vi "Teleop.vi"(10 "Match Info":T1={"Autonomous Elapsed Seconds"=0.0, "TeleOp Elapsed Seconds"=0.0, "Disabled Elapsed Seconds"=0.0, "Visited Autonomous"=FALSE, "Visited TeleOp"=FALSE, "Visited Disabled"=FALSE, "Autonomous Settings"={"Autonomous Style"=enum."Independent", "VI Refnum"=refnum}}, 11 "Call Context":T2=enum."Stop") -> ()   [LabVIEW 2018]
doc: "This VI is called for each enabled TeleOp packet received from the DS. It is typically used to read from joysticks and other inputs and update I/O or setpoints for timed control loops. It should complete and return within 20 milliseconds or risk missing DS packets."
uses:
  <vilib>/Rock Robotics/WPI/DriverStation/WPI_DriverStationDerivedRobotMode.ctl
  <vilib>/Rock Robotics/WPI/DriverStation/WPI_DriverStationMatch Info.ctl
  Typedef/XBox Axis.ctl
  Typedef/XBox Buttons.ctl
  <vilib>/Rock Robotics/WPI/Utilities/WPI_GetSetVariantRefNum.vi
  <vilib>/Rock Robotics/Network Tables/NT Write Boolean Array.vi
  <vilib>/Rock Robotics/Network Tables/NT Write Numeric Array.vi
  <vilib>/Rock Robotics/Network Tables/NT Write Number.vi
  <vilib>/Rock Robotics/Network Tables/NT Read Number.vi
  Subsystem Sequencer/Commands/Elevator to Position.vi
  <vilib>/Rock Robotics/WPI/MotorControl/WPI_MotorControlRefNum Registry Get.vi
  <vilib>/Rock Robotics/WPI/ThirdParty/REV Robotics/SPARK MAX/SubVI/Public/Spark MAX Set Smart Motion Constraints.vi
  <vilib>/Rock Robotics/WPI/Solenoid/WPI_SolenoidRefNum Registry Get.vi
  <vilib>/Rock Robotics/WPI/Solenoid/WPI_SolenoidSet.vi
  <vilib>/Rock Robotics/WPI/Solenoid/WPI_SolenoidSetEnum.vi
  Drive/CAN Functions/CAN 6 SPARK MAX Motor Ref Get.vi
  Drive/CAN Functions/CAN 6 SPARK MAX Motor Set Idle Modes.vi
  Subsystem Sequencer/Commands/Climb Sequence Three.vi
  Subsystem Sequencer/Commands/Climb Sequence Two.vi
  Subsystem Sequencer/Commands/Climb Sequence One.vi
panel:
  in  "max queso power (1)":dbl=0.6
  in  "Limelight Speed Limit":dbl=0.5
  in  "Elevator Slow Acceleration":dbl=800.0
  in  "Elevator Slow Velocity":dbl=400.0
  in  "Arm angle from 'Y'":dbl=86.0 format="%#_13g"
  in  "Joystick Deadband":dbl=0.06 format="%#_13g"
  in  "Throttle Sensitivity":dbl(slide)=0.7142857142857142 scale=0.0..1.0
  in  "Elevator Speed":dbl=1.5 format="%#_13g"
  in  "QuesoTurn Sensitivty":dbl=0.7
  in  "Cheesy Sensitivity":dbl(slide)=0.5864661654135338 scale=0.0..1.0
  in  "Arcade to Queso":bool=TRUE
  # "<-- This is not motor speed!"
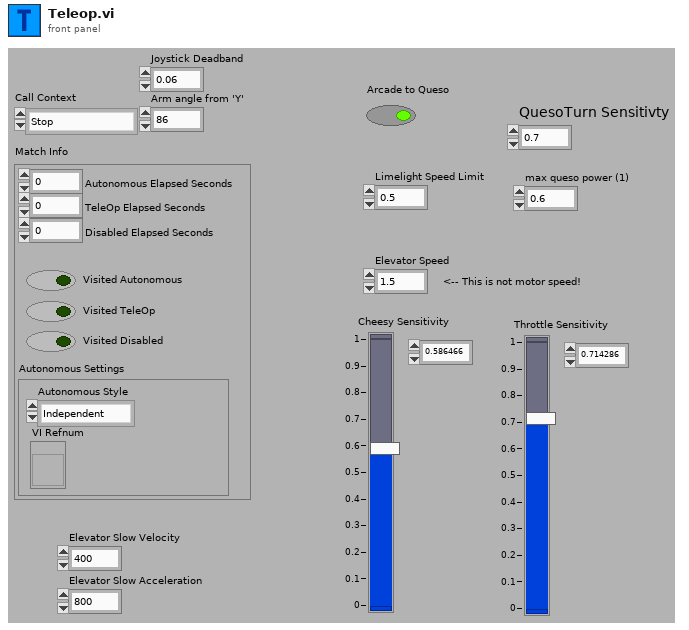
[diagram p1: front panel]
types:
  T1 = typedef "WPI_DriverStationMatch Info.ctl" = cluster{"Autonomous Elapsed Seconds":dbl, "TeleOp Elapsed Seconds":dbl, "Disabled Elapsed Seconds":dbl, "Visited Autonomous":bool, "Visited TeleOp":bool, "Visited Disabled":bool, "Autonomous Settings":cluster{"Autonomous Style":enum16{"Iterative", "Independent"}, "VI Refnum":refnum<vi>}}
  T2 = typedef "WPI_DriverStationDerivedRobotMode.ctl" = enum16{"Init", "Execute", "Stop"}
  T3 = typedef "XBox Buttons.ctl" = enum16{"A", "B", "X", "Y", "Left Bumper", "Right Bumper", "Back", "Start", "Left Joystick", "Right Joystick"}
  T4 = typedef "XBox Axis.ctl" = enum16{"Left X", "Left Y", "Left Trigger", "Right Trigger", "Right X", "Right Y"}
  T5 = typedef "WPI_JoystickDevRef.ctl" = cluster{"Device":T6}
  T6 = typedef "WPI_JoystickDeviceEnum.ctl" = enum16{"USB 0", "USB 1", "USB 2", "USB 3", "USB 4", "USB 5"}
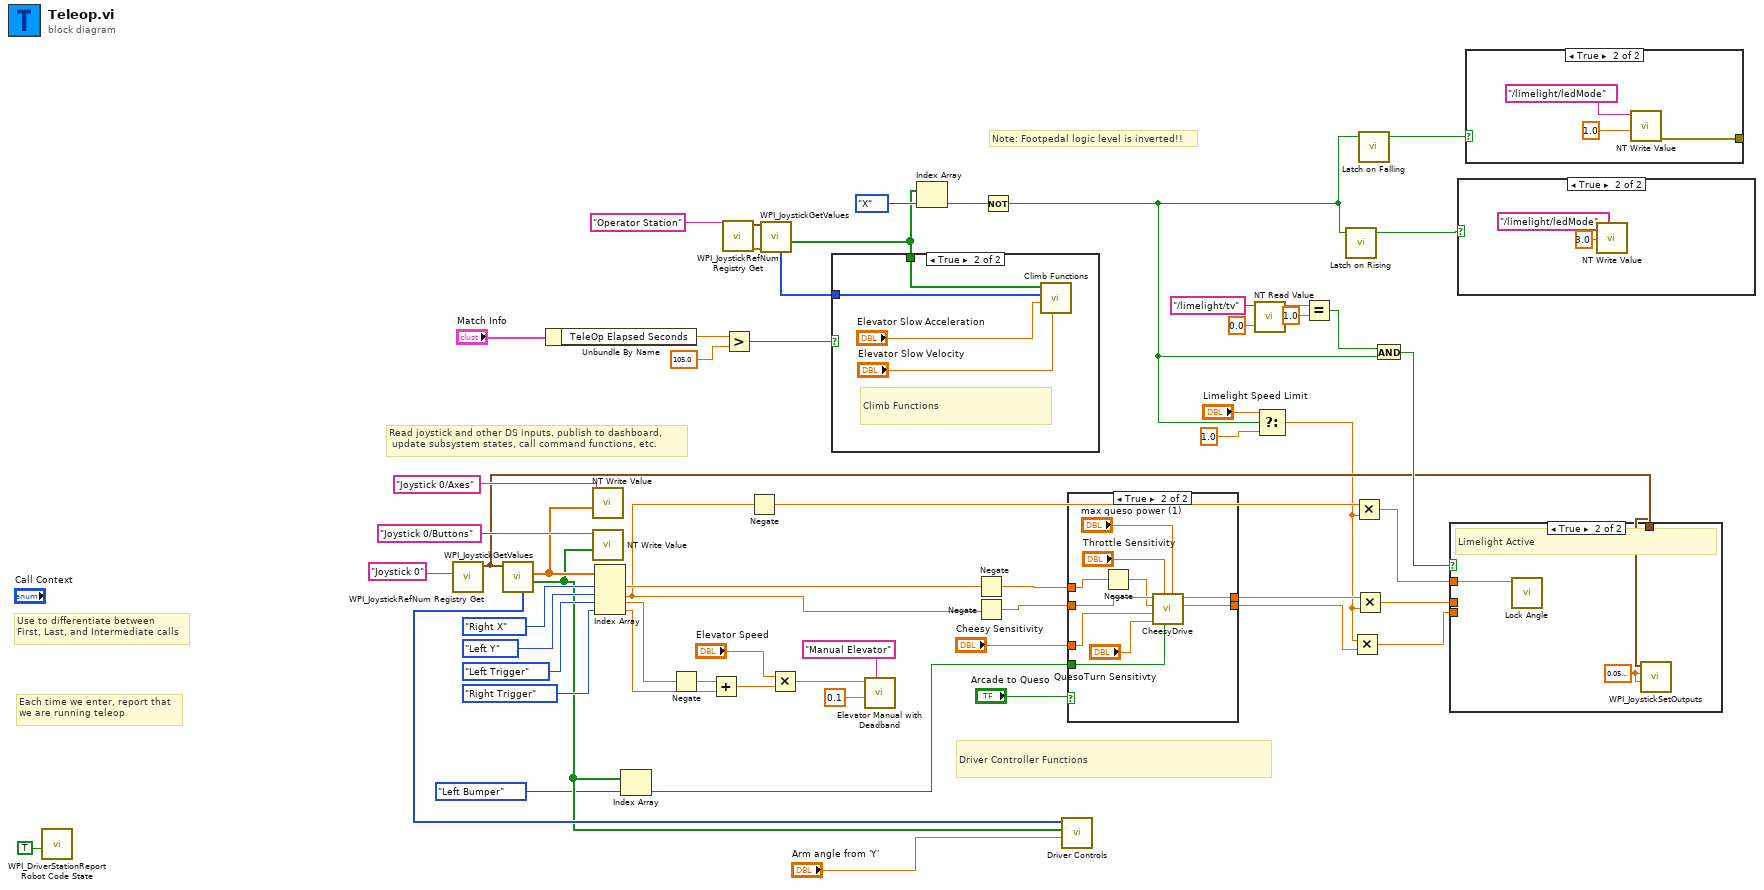
[diagram p0: block diagram]
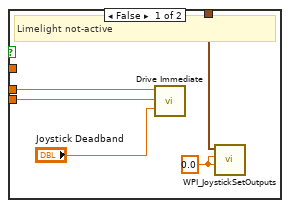
[diagram p5: hidden frame]
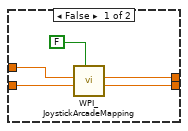
[diagram p6: hidden frame]
diagram:
  # "Driver Controller Functions"
  # "Note: Footpedal logic level is inverted!!"
  # "Read joystick and other DS inputs, publish to dashboard,\n update subsystem states, call command functions, etc."
  # "Each time we enter, report that\nwe are running teleop"
  # "Use to differentiate between\nFirst, Last, and Intermediate calls"
  n1 = call <vilib>:"WPI_DriverStationReport Robot Code State.vi"("TeleOp"=TRUE ("Autonomous")) -> ()  [unwired: 10 in, 1 out]
  n2 = call <vilib>:"WPI_JoystickRefNum Registry Get.vi"("refnum name"="Joystick 0") -> ("JoystickDevRef"=w24:T5)  [unwired: 1 in, 9 out]
  n3 = call <vilib>:"WPI_JoystickGetValues.vi"("JoystickDevRef"=w24) -> ("Buttons"=w17:bool[], "Axes"=w54:dbl[], "POVs"=w19:i16[])  [unwired: 6 in, 2 out]
  n4 = Unbundle By Name("Match Info") -> ("TeleOp Elapsed Seconds"=w3:dbl)
  n5 = call-poly <vilib>:"NT Write Value.vi"("Numeric Array"=w54, "Name"="Joystick 0/Axes") -> ()  [unwired: 9 in, 1 out]
  n6 = call-poly <vilib>:"NT Write Value.vi"("Boolean Array"=w17, "Name"="Joystick 0/Buttons") -> ()  [unwired: 9 in, 1 out]
  n7 = Index Array(array=w54, index #1=XBox_Axis."Right X" ("Enum"), index #2=XBox_Axis."Left Y" ("Enum"), index #3=XBox_Axis."Left Trigger" ("Enum"), index #4=XBox_Axis."Right Trigger" ("Enum")) -> (element #1=w50:dbl, element #2=w23:dbl, element #3=w43:dbl, element #4=w42:dbl)
  n8 = Index Array(array=w17, index=XBox_Buttons."Left Bumper" ("Enum")) -> (element=w15:bool)
  n9 = Negate(x=w43) -> (-x=w40:dbl)
  n10 = Add(x=w40, y=w42) -> (x+y=w41:dbl)
  n11 = call <vilib>:"WPI_JoystickRefNum Registry Get.vi"("refnum name"="Operator Station") -> ("error out"=w35:errorcluster, "JoystickDevRef"=w34:T5)  [unwired: 9 in]
  n12 = Greater?(x=w3, y=105.0) -> (0:w2:bool)
  n13 = Negate(x=w23) -> (-x=w8:dbl)
  n14 = call <vilib>:"WPI_JoystickGetValues.vi"("error in (no error)"=w35, "JoystickDevRef"=w34) -> ("Buttons"=w18:bool[], "POVs"=w20:i16[])  [unwired: 5 in, 3 out]
  n15 = Multiply(x="Elevator Speed", y=w41) -> (x*y=w38:dbl)
  n16 = case shown="True" w2 {
    tunnel: w20 -> [_ w62]
    tunnel: w18 -> [_ w61]
    frame False {
    }
    frame True {
      # "Climb Functions"
      n17 = call "Climb Functions.vi"("Elevator Slow Velocity"="Elevator Slow Velocity", "Elevator Slow Acceleration"="Elevator Slow Acceleration", "POVs"=w62, "Buttons"=w61) -> ()  [unwired: 8 in]
    }
  }
  n18 = call "Elevator Manual with Deadband.vi"("Description"="Manual Elevator", "Deadband Value"=0.1, "Setpoint"=w38) -> ()  [unwired: 8 in, 1 out]
  n19 = Index Array(array=w18, index=XBox_Buttons."X" ("Enum")) -> (element=w31:bool)
  n20 = Negate(x=w50) -> (-x=w48:dbl)
  n21 = Negate(x=w23) -> (-x=w49:dbl)
  n22 = Not(x=w31) -> (.not. x?=w7:bool)
  n23 = call "Driver Controls.vi"("Arm angle from 'Y'"="Arm angle from 'Y'", "Buttons"=w17, "POVs"=w19) -> ()  [unwired: 9 in]
  n24 = case shown="True" "Arcade to Queso" {
    tunnel: w49 -> [w66 w74]
    tunnel: w48 -> [w67 w73]
    tunnel: [w65 w77] -> w12
    tunnel: [w64 w76] -> w10
    tunnel: w15 -> [_ w75]
    tunnel: "Cheesy Sensitivity" -> [_ w71]
    frame False {
      n25 = call <vilib>:"WPI_JoystickArcadeMapping.vi"("Square Inputs"=FALSE, "Y axis value"=w66, "X axis value"=w67) -> ("Right Motor Value"=w65:dbl, "Left Motor Value"=w64:dbl)  [unwired: 7 in]
    }
    frame True {
      n26 = Negate(x=w73) -> (-x=w72:dbl)
      n27 = call "CheesyDrive.vi"("max queso power (1)"="max queso power (1)", "Quickturn"=w75, "Throttle Sensitivity"="Throttle Sensitivity", "QuickTurn Sensitivty"="QuesoTurn Sensitivty", "Queso Arc Sensitivty"=w71, "Wheel"=w72, "Throttle"=w74) -> ("Right PWM"=w77:dbl, "Left PWM"=w76:dbl)  [unwired: 3 in]
    }
  }
  n28 = call-poly <vilib>:"NT Read Value.vi"("Default Value"=0.0, "Name"="/limelight/tv") -> ("Numeric"=w28:dbl)  [unwired: 8 in, 1 out]
  n29 = Select(t="Limelight Speed Limit", s=w7, f=1.0) -> (s? t:f=w5:dbl)
  n30 = Equal?(x=w28, y=1.0) -> (x = y?=w26:bool)
  n31 = call "Latch on Rising.vi"("Boolean in"=w7) -> ("Boolean out"=w22:bool)  [unwired: 4 in]
  n32 = Multiply(x=w5, y=w12) -> (x*y=w13:dbl)
  n33 = Multiply(x=w8, y=w5) -> (x*y=w9:dbl)
  n34 = Multiply(x=w10, y=w5) -> (x*y=w11:dbl)
  n35 = call "Latch on Falling.vi"("Boolean in"=w7) -> ("Boolean out"=w21:bool)  [unwired: 4 in]
  n36 = And(x=w26, y=w7) -> (x .and. y?=w25:bool)
  n37 = case shown="True" w25 {
    tunnel: w13 -> [w81 _]
    tunnel: w11 -> [w80 _]
    tunnel: w9 -> [_ w85]
    tunnel: w24 -> [w79 w84]
    frame False {
      w78 = sgl 0.0 ("Right Rumble")
      # "Limelight not-active"
      n38 = call "Drive Immediate.vi"("Deadband Value"="Joystick Deadband", "Right Setpoint"=w81, "Left Setpoint"=w80) -> ()  [unwired: 8 in, 1 out]
      n39 = call <vilib>:"WPI_JoystickSetOutputs.vi"("Right Rumble"=w78, "Left Rumble"=w78, "JoystickDevRef"=w79) -> ()  [unwired: 7 in, 2 out]
    }
    frame True {
      w83 = sgl 0.05 ("Left Rumble")
      # "Limelight Active"
      n40 = call "Lock Angle.vi"("Setpoint"=w85) -> ()  [unwired: 11 in]
      n41 = call <vilib>:"WPI_JoystickSetOutputs.vi"("Right Rumble"=w83, "Left Rumble"=w83, "JoystickDevRef"=w84) -> ()  [unwired: 7 in, 2 out]
    }
  }
  n42 = case shown="True" w22 {
    frame False {
    }
    frame True {
      n43 = call-poly <vilib>:"NT Write Value.vi"("Numeric"=3.0, "Name"="/limelight/ledMode") -> ()  [unwired: 9 in, 1 out]
    }
  }
  n44 = case shown="True" w21 {
    tunnel: [_ w88] -> _
    frame False {
    }
    frame True {
      n45 = call-poly <vilib>:"NT Write Value.vi"("Numeric"=1.0, "Name"="/limelight/ledMode") -> ("error out"=w88:errorcluster)  [unwired: 9 in]
    }
  }
